vi "GOOPUtil_IsEmptyObject.vi"(1 "LabVIEW Object":refnum<class>) -> (0 "IsEmpty?":bool)   [LabVIEW 2016, in "GOOPUtility.lvlib"]
uses:
  <vilib>/addons/GOOPUtility/GOOPUtility.lvlib
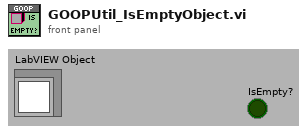
[diagram p1: front panel]
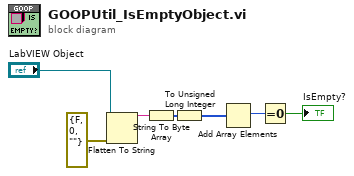
[diagram p0: block diagram]
diagram:
  n1 = Flatten To String(anything="LabVIEW Object", error in (no error)=errorcluster {"status"=FALSE, "code"=0, "source"=""}) -> (data string=w7:string)  [unwired: 2 in, 2 out]
  n2 = String To Byte Array(string=w7) -> (unsigned byte array=w6:u8[])
  n3 = To Unsigned Long Integer(number=w6) -> (unsigned 32bit integer=w1:u32[])
  n4 = Add Array Elements(numeric array=w1) -> (sum=w5:u32)
  n5 = Equal To 0?(x=w5) -> (x = 0?=→"IsEmpty?":bool)
